vi "Main Page GUID.vi"() -> (3 "Main Page GUID":string="37c56d03-17da-482b-8988-568955beadf2")   [LabVIEW 2020, in "DSF Shared.lvlib"]
uses:
  DSF Shared.lvlib
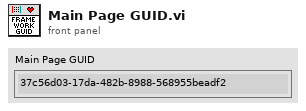
[diagram p1: front panel]
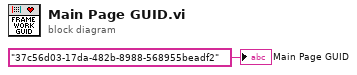
[diagram p0: block diagram]
diagram:
  "Main Page GUID" <- "37c56d03-17da-482b-8988-568955beadf2" ("Data Sharing Framework")
